vi "Load File.vi"(8 "error in":errorcluster, 10 "File Path":path, 11 "EDS Viewer in":refnum<class "EDS Viewer.lvclass">) -> (0 "error out":errorcluster, 3 "EDS Viewer out":refnum<class "EDS Viewer.lvclass">)   [LabVIEW 2024, in "EDS Viewer.lvlib" / "EDS Viewer.lvclass"]
uses:
  EDS Viewer.lvclass
  EDS Viewer.lvclass/EDS Viewer.ctl
  <vilib>/Utility/config.llb/Read Key (String).vi
  <vilib>/Utility/config.llb/NI_LVConfig.lvlib
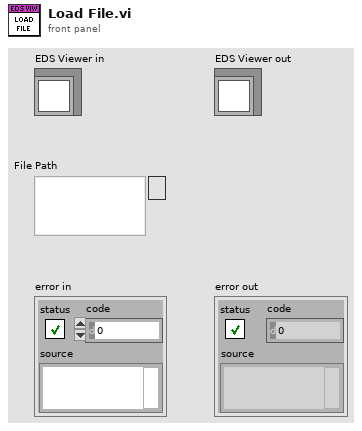
[diagram p1: front panel]
types:
  T1 = typedef "NI_LVConfig.lvlib/Config Data RefNum.ctl" = refnum<k1>
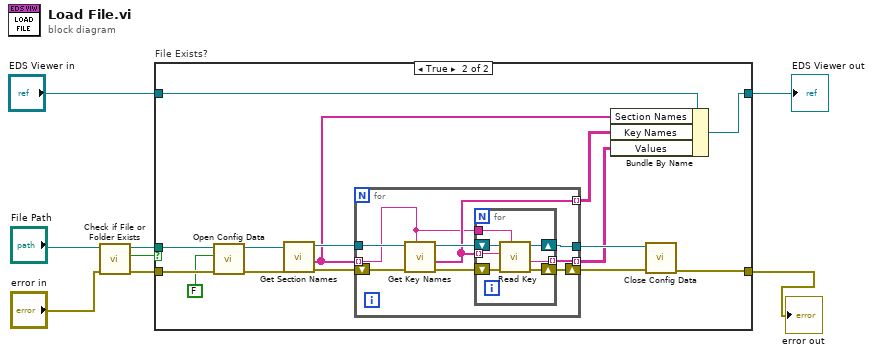
[diagram p0: block diagram]
diagram:
  n1 = call <vilib>:"Check if File or Folder Exists.vi"("error in (no error)"="error in", "path"="File Path") -> ("error out"=w4:errorcluster, "file or folder exists?"=w6:bool, "dup path"=w5:path)  [unwired: 7 in]
  n2 = case "File Exists?" shown="True" w6 {
    tunnel: w5 -> [_ w25]
    tunnel: w4 -> [w10 w24]
    tunnel: [w10 w17] -> w3
    tunnel: "EDS Viewer in" -> [w9 w14]
    tunnel: [w9 w13] -> w1
    frame False {
    }
    frame True {
      n3 = call <vilib>:"Open Config Data.vi"("error in (no error)"=w24, "create file if necessary (T)"=FALSE, "configuration file path"=w25) -> ("error out"=w22:errorcluster, "refnum"=w21:T1)  [unwired: 6 in, 1 out]
      n4 = call <vilib>:"Get Section Names.vi"("error in (no error)"=w22, "refnum"=w21) -> ("error out"=w20:errorcluster, "section names"=w12:string[], "refnum out"=w19:T1)  [unwired: 7 in]
      n5 = for {
        tunnel: w12 -> [w27] mode=indexing
        shift-right: [w31] -> w18
        shift-left: w20 -> [w34]
        tunnel: w19 -> [w33]
        tunnel: [w28] -> w15 mode=indexing
        tunnel: [w29] -> w16
        tunnel: [w26] -> w11 mode=indexing
        n6 = call <vilib>:"Get Key Names.vi"("section"=w27, "error in (no error)"=w34, "refnum"=w33) -> ("error out"=w32:errorcluster, "key names"=w28:string[], "refnum out"=w30:T1)  [unwired: 5 in, 1 out]
        n7 = for {
          shift-right: [w40] -> w31
          shift-left: w32 -> [w41]
          shift-right: [w38] -> w29
          shift-left: w30 -> [w39]
          tunnel: w28 -> [w37] mode=indexing
          tunnel: w27 -> [w36]
          tunnel: [w35] -> w26 mode=indexing
          n8 = call-poly <vilib>:"Read Key.vi"("section"=w36, "error in (no error)"=w41, "key"=w37, "refnum"=w39) -> ("error out"=w40:errorcluster, "value"=w35:string, "refnum out"=w38:T1)  [unwired: 4 in, 1 out]
        }
      }
      n9 = Bundle By Name(cluster=w14, "Section Names"=w12, "Key Names"=w15, "Values"=w11) -> (w13:refnum<class "EDS Viewer.lvclass">)
      n10 = call <vilib>:"Close Config Data.vi"("error in (no error)"=w18, "refnum"=w16) -> ("error out"=w17:errorcluster)  [unwired: 8 in, 1 out]
    }
  }
  "error out" <- w3
  "EDS Viewer out" <- w1
